vi "sub_SDR_mimo_tx.vi"(6 "Init Tx Buffer":bool, 7 "System options":T1, 10 "Packets":string[](array[string])) -> (0 "Link occupation [%]":dbl, 1 "Tx Buffer size":i32, 2 "Tx Frame":cdb[][](array[numeric]), 3 "Ok?":bool)   [LabVIEW 2012]
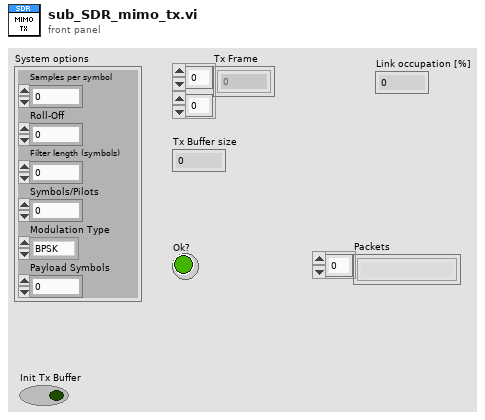
[diagram p1: front panel]
types:
  T1 = cluster{"Samples per symbol":i32, "Roll-Off":dbl, "Filter length (symbols)":i32, "Symbols/Pilots":i32, "Modulation Type":enum16{"BPSK", "4-QAM", "16-QAM", "64-QAM"}, "Payload Symbols":i32}
  T2 = cluster{"Samples per symbol":i32, "Roll-Off":dbl, "Filter length (symbols)":i32}
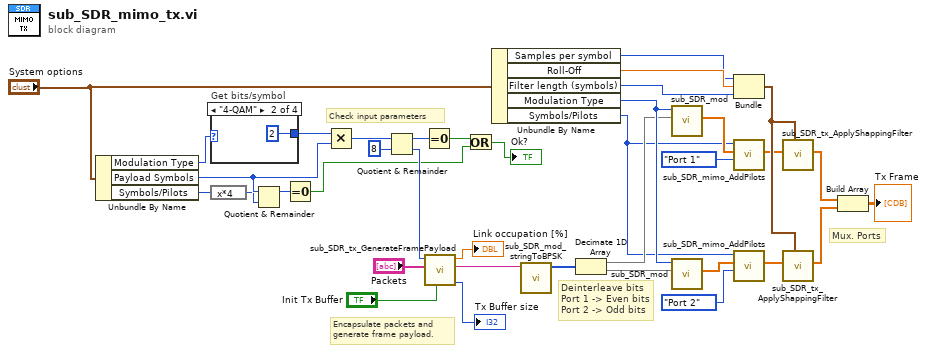
[diagram p0: block diagram]
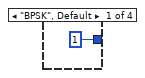
[diagram p2: hidden frame]
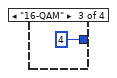
[diagram p3: hidden frame]
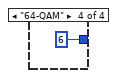
[diagram p4: hidden frame]
diagram:
  # "Deinterleave bits\nPort 1 -> Even bits\nPort 2 -> Odd bits"
  # "Mux. Ports"
  # "Encapsulate packets and\ngenerate frame payload."
  # "Check input parameters"
  n1 = Unbundle By Name("System options") -> ("Modulation Type"=w32:enum16{"BPSK", "4-QAM", "16-QAM", "64-QAM"}, "Payload Symbols"=w18:i32, "Symbols/Pilots"=w7:i32)
  n2 = case "Get bits/symbol" shown="\"4-QAM\"" w32 {
    tunnel: [1 2 4 6] -> w33
    frame "BPSK", Default {
    }
    frame "4-QAM" {
    }
    frame "16-QAM" {
    }
    frame "64-QAM" {
    }
  }
  n3 = expression code="x*4"(w7) -> (w17:i32)
  n4 = Quotient & Remainder(x=w18, y=w17) -> (x-y*floor(x/y)=w16:i32)  [unwired: 1 out]
  n5 = Equal To 0?(x=w16) -> (x = 0?=w13:bool)
  n6 = Multiply(x=w33, y=w18) -> (x*y=w35:i32)
  n7 = Quotient & Remainder(x=w35, y=8) -> (x-y*floor(x/y)=w37:i32, floor(x/y)=w36:i32)
  n8 = Equal To 0?(x=w37) -> (x = 0?=w14:bool)
  n9 = call "sub_SDR_tx_GenerateFramePayload.vi"("Init?"="Init Tx Buffer", "Packets"="Packets", "Payload Length"=w36) -> ("Buffer Length"=→"Tx Buffer size":i32, "Payload String"=w21:string, "Link occupation [%]"=→"Link occupation [%]":dbl)  [unwired: 6 in]
  n10 = Or(x=w14, y=w13) -> (x .or. y?=→"Ok?":bool)
  n11 = Unbundle By Name("System options") -> ("Samples per symbol"=w27:i32, "Roll-Off"=w28:dbl, "Filter length (symbols)"=w29:i32, "Modulation Type"=w8:enum16{"BPSK", "4-QAM", "16-QAM", "64-QAM"}, "Symbols/Pilots"=w1:i32)
  n12 = call "sub_SDR_mod_stringToBPSK.vi"("Input String"=w21) -> ("Array"=w22:i16[])  [unwired: 10 in]
  n13 = Decimate 1D Array ("Deinterleave bits")(w22) -> (w3:i16[], w2:i16[])
  n14 = call "sub_SDR_mod.vi"("Array"=w3, "Modulation Type"=w8) -> ("Array out"=w24:cdb[])  [unwired: 9 in]
  n15 = call "sub_SDR_mod.vi"("Array"=w2, "Modulation Type"=w8) -> ("Array out"=w12:cdb[])  [unwired: 9 in]
  n16 = Bundle("Samples per symbol"=w27, "Roll-Off"=w28, "Filter length (symbols)"=w29) -> (w30:T2)  [unwired: 1 in]
  n17 = call "sub_SDR_mimo_AddPilots.vi"("Port"=enum16{"Port 1", "Port 2"}."Port 1", "Array in"=w24, "Symbols/Pilots"=w1) -> ("Array Out"=w26:cdb[])  [unwired: 8 in]
  n18 = call "sub_SDR_mimo_AddPilots.vi"("Port"=enum16{"Port 1", "Port 2"}."Port 2", "Array in"=w12, "Symbols/Pilots"=w1) -> ("Array Out"=w11:cdb[])  [unwired: 8 in]
  n19 = call "sub_SDR_tx_ApplyShappingFilter.vi"("Filter Options"=w30, "Data Symbols"=w26) -> ("Shaped symbols"=w6:cdb[])  [unwired: 9 in]
  n20 = call "sub_SDR_tx_ApplyShappingFilter.vi"("Filter Options"=w30, "Data Symbols"=w11) -> ("Shaped symbols"=w5:cdb[])  [unwired: 9 in]
  n21 = Build Array(w6, w5) -> (→"Tx Frame":cdb[][])
